vi "(Un)Deploy ABORT.vi"(6 "Undeploy?":bool, 8 "error in (no error)":errorcluster) -> (0 "error out":errorcluster)   [LabVIEW 2020, in "TALOS.lvlib"]
uses:
  TALOS.lvlib
  Global Constants.vi
  Is in Packed Library.vi
  TALOS Root path.vi
  Classes/Circus Shared Variables/Circus Shared Variables.lvclass
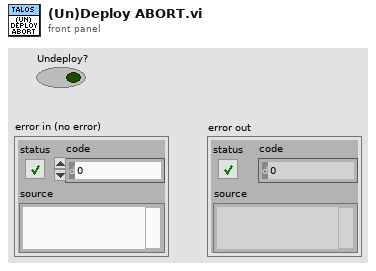
[diagram p1: front panel]
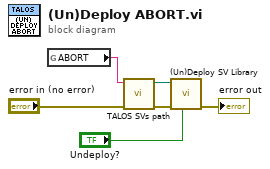
[diagram p0: block diagram]
diagram:
  n1 = global read "Global Constants.vi" "ABORT"() -> (w1:string)
  n2 = call "TALOS SVs path.vi"("error in (no error)"="error in (no error)", "Library Name"=w1) -> ("error out"=w3:errorcluster, "Library path"=w4:path)  [unwired: 8 in]
  n3 = call "(Un)Deploy SV Library.vi"("Undeploy?"="Undeploy?", "error in (no error)"=w3, "Library path"=w4) -> ("error out"=→"error out":errorcluster)  [unwired: 8 in]
